vi "UpdateRequestName.vi"(7 "NameType":enum16{"StartName", "AckName", "FulfilledName"}(ring), 8 "error in":errorcluster, 9 "Name":string, 10 "RequestID":u32) -> (0 "error out":errorcluster)   [LabVIEW 2015, in "DatabaseApi.lvlib"]
uses:
  DatabaseApi.lvlib
  TypeDef/Request/RequestsTableColumnNamesRing.ctl
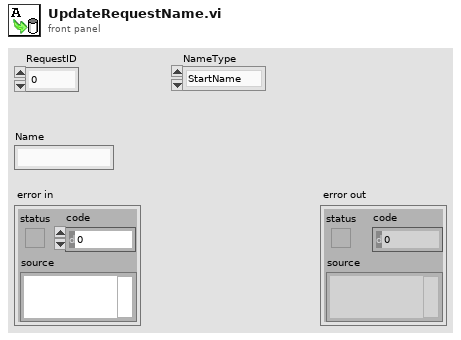
[diagram p1: front panel]
types:
  T1 = typedef "DatabaseApi.lvlib/RequestsTableColumnNamesRing.ctl" = enum16{"RequestID", "PersonnelType", "StartTime", "StartName", "AckTime", "AckName", "FulfilledTime", "FulfilledName", "Description"}
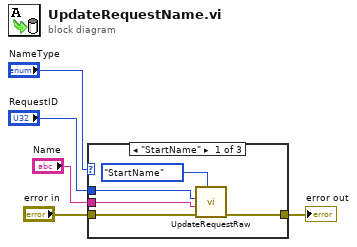
[diagram p0: block diagram]
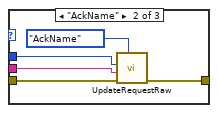
[diagram p2: hidden frame]
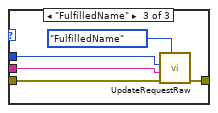
[diagram p3: hidden frame]
diagram:
  n1 = case shown="\"StartName\"" "NameType" {
    tunnel: "error in" -> [w10 w15 w20]
    tunnel: "RequestID" -> [w9 w14 w19]
    tunnel: [w8 w13 w18] -> w3
    tunnel: "Name" -> [w6 w11 w16]
    frame "StartName" {
      n2 = call "UpdateRequestRaw.vi"("Data to update"=RequestsTableColumnNamesRing."StartName", "error in"=w10, "data"=w6, "RequestID"=w9) -> ("error out"=w8:errorcluster)  [unwired: 7 in]
    }
    frame "AckName" {
      n3 = call "UpdateRequestRaw.vi"("Data to update"=RequestsTableColumnNamesRing."AckName", "error in"=w15, "data"=w11, "RequestID"=w14) -> ("error out"=w13:errorcluster)  [unwired: 7 in]
    }
    frame "FulfilledName" {
      n4 = call "UpdateRequestRaw.vi"("Data to update"=RequestsTableColumnNamesRing."FulfilledName", "error in"=w20, "data"=w16, "RequestID"=w19) -> ("error out"=w18:errorcluster)  [unwired: 7 in]
    }
  }
  "error out" <- w3
